vi "Clamp Load.vi"() -> (3 "End":bool)   [LabVIEW 2013]
doc: "This VI is used in 2-ball Autonomous Mode in order to load the second ball onto the robot."
uses:
  <vilib>/Rock Robotics/WPI/Solenoid/Deprecated/WPI_SolenoidSetBool.vi
panel:
  out "State":enum16{"Clamp Up", "Clamp Open", "Clamp Down"}(ring)
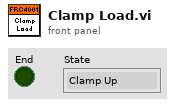
[diagram p1: front panel]
types:
  T1 = typedef "WPI_DigitalInputDevRef.ctl" = cluster{"DevStatus":errorcluster, "DIO Channel":T2, "Digital Module":T3}
  T2 = typedef "FPGA_DIOChannel.ctl" = enum8{"DIO 1", "DIO 2", "DIO 3", "DIO 4", "DIO 5", "DIO 6", "DIO 7", "DIO 8", "DIO 9", "DIO 10", "DIO 11", "DIO 12", "DIO 13", "DIO 14", "Invalid"}
  T3 = typedef "FPGA_TypedefDigitalModule.ctl" = enum16{"Digital Module 1", "Digital Module 2"}
  T4 = typedef "WPI_MotorControlDeviceRef.ctl" = cluster{"DeviceStatus":errorcluster, "Type":enum16{"PWM", "CAN"}, "PWM":cluster{"Digital Module":T3, "PWM Channel":T5, "DeadBand":T6}, "CAN":cluster{"Device Number":u8, "Control Mode":T7, "Semaphore":T8, "Max Vout":dbl}, "Invert":bool, "TransformRef":T9, "InvTransformRef":T9}
  T5 = typedef "FPGA_DIOPWMChannel.ctl" = enum8{"PWM 1", "PWM 2", "PWM 3", "PWM 4", "PWM 5", "PWM 6", "PWM 7", "PWM 8", "PWM 9", "PWM 10", "Invalid"}
  T6 = typedef "WPI_PWMDeadband.ctl" = cluster{"Name":string, "maxPositivePwm":i32, "minPositivePwm":i32, "centerPwm":i32, "maxNegativePwm":i32, "minNegativePwm":i32, "angularRange":u16}
  T7 = typedef "WPI_CANJaguar_ControlMode.ctl" = enum8{"Percent VBus", "Current", "Speed", "Position", "Voltage"}
  T8 = typedef "Semaphore RefNum" = refnum<k1>
  T9 = typedef "WPI_PWMTransform_ConPane.ctl" = refnum<vi>
  T10 = typedef "WPI_SolenoidDevRef.ctl" = cluster{"DevStatus":errorcluster, "Solenoid Module":T11, "Forward Solenoid Channel":T12, "Reverse Solenoid Channel":T12}
  T11 = typedef "FPGA_TypedefSolenoidModule.ctl" = enum16{"Solenoid Module 1", "Solenoid Module 2"}
  T12 = typedef "WPI_SolenoidChannel.ctl" = enum8{"Solenoid 1", "Solenoid 2", "Solenoid 3", "Solenoid 4", "Solenoid 5", "Solenoid 6", "Solenoid 7", "Solenoid 8", "Invalid"}
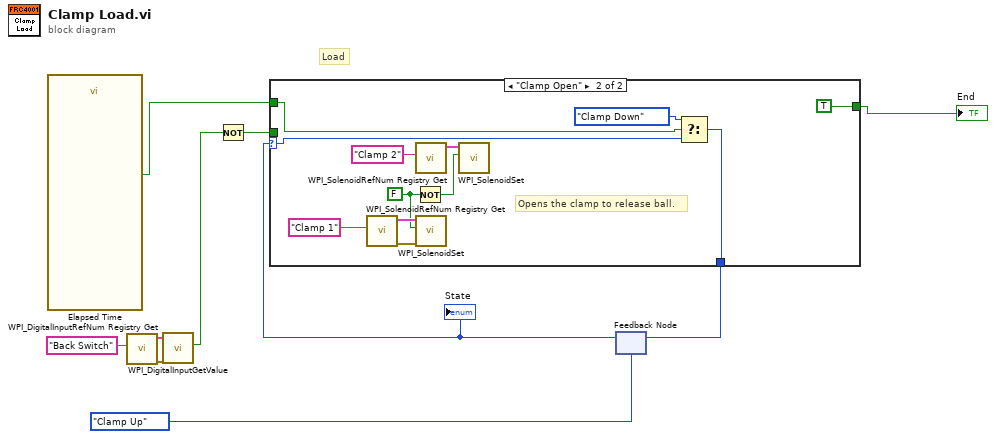
[diagram p0: block diagram]
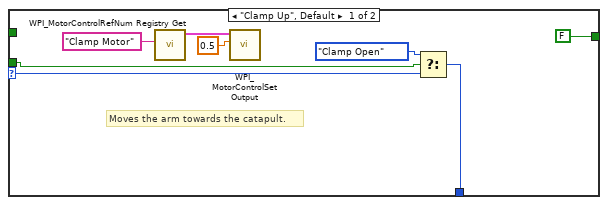
[diagram p2: hidden frame]
diagram:
  # "Load"
  n1 = call "Elapsed Time"() -> ("Time has Elapsed"=w6:bool)  [unwired: 12 in, 7 out]
  n2 = call <vilib>:"WPI_DigitalInputRefNum Registry Get.vi"("refnum name"="Back Switch") -> ("error out"=w4:errorcluster, "DigitalInputDevRef"=w3:T1)  [unwired: 9 in]
  n3 = call <vilib>:"WPI_DigitalInputGetValue.vi"("error in (no error)"=w4, "DigitalInputDevRef"=w3) -> ("Value"=w2:bool)  [unwired: 7 in, 2 out]
  n4 = Not(x=w2) -> (.not. x?=w1:bool)
  n5 = feedback #1(enum16{"Clamp Up", "Clamp Open", "Clamp Down"}."Clamp Up") -> (w8:enum16{"Clamp Up", "Clamp Open", "Clamp Down"})
  "State" <- w8
  n6 = case shown="\"Clamp Open\"" w8 {
    selector: w8 -> [w18 w30]
    tunnel: [w16 w28] -> w9
    tunnel: [FALSE TRUE] -> w7
    tunnel: w6 -> [_ w19]
    tunnel: w1 -> [w11 _]
    frame "Clamp Up", Default {
      # "Moves the arm towards the catapult."
      n7 = call <vilib>:"WPI_MotorControlRefNum Registry Get.vi"("refnum name"="Clamp Motor") -> ("MotorControlDevRef"=w13:T4)  [unwired: 9 in, 1 out]
      n8 = call <vilib>:"WPI_MotorControlSetOutput.vi"("Output"=0.5, "MotorControlDevRef"=w13) -> ()  [unwired: 7 in, 3 out]
      n9 = Select(t=enum16{"Clamp Up", "Clamp Open", "Clamp Down"}."Clamp Open", s=w11, f=w18) -> (s? t:f=w16:enum16{"Clamp Up", "Clamp Open", "Clamp Down"})
    }
    frame "Clamp Open" {
      w23 = FALSE
      # "Opens the clamp to release ball."
      n10 = call <vilib>:"WPI_SolenoidRefNum Registry Get.vi"("refnum name"="Clamp 1") -> ("error out"=w24:errorcluster, "SolenoidDevRef"=w25:T10)  [unwired: 9 in]
      n11 = Not(x=w23) -> (.not. x?=w21:bool)
      n12 = call <vilib>:"WPI_SolenoidRefNum Registry Get.vi"("refnum name"="Clamp 2") -> ("SolenoidDevRef"=w22:T10)  [unwired: 9 in, 1 out]
      n13 = call-poly <vilib>:"WPI_SolenoidSet.vi"("error in (no error)"=w24, "Value"=w23, "SolenoidDevRef"=w25) -> ()  [unwired: 7 in, 2 out]
      n14 = call-poly <vilib>:"WPI_SolenoidSet.vi"("Value"=w21, "SolenoidDevRef"=w22) -> ()  [unwired: 8 in, 2 out]
      n15 = Select(t=enum16{"Clamp Up", "Clamp Open", "Clamp Down"}."Clamp Down", s=w19, f=w30) -> (s? t:f=w28:enum16{"Clamp Up", "Clamp Open", "Clamp Down"})
    }
  }
  "End" <- w7
  n16 = feedback-in #1(w9) -> ()
